vi "SetChainLength.vi"(8 "error in (no error)":errorcluster, 10 "Chain Length":u8, 11 "ControlState in":T1 {"ChainMask" format="0x%02x"}) -> (0 "error out":errorcluster, 3 "ControlState out":T1 {"ChainMask" format="0x%02x"})   [LabVIEW 2020, in "ArduinoSerialBling.lvlib"]
uses:
  ArduinoSerialBling.lvlib
  ControlState.ctl
  ChainState.ctl
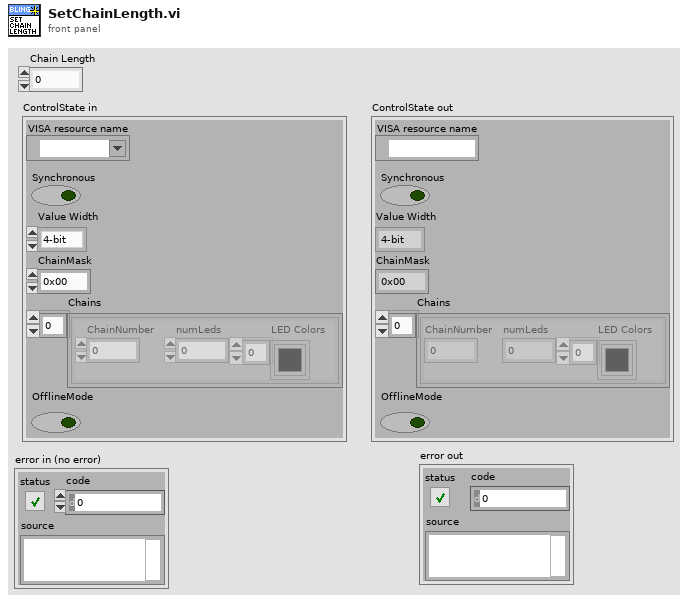
[diagram p1: front panel]
types:
  T1 = typedef "ArduinoSerialBling.lvlib/ControlState.ctl" = cluster{"VISA resource name":refnum<visa-resource-name>, "Synchronous":bool, "Value Width":enum16{"4-bit", "8-bit"}, "ChainMask":u8, "Chains":T2[], "OfflineMode":bool}
  T2 = typedef "ArduinoSerialBling.lvlib/ChainState.ctl" = cluster{"ChainNumber":u8, "numLeds":u8, "LED Colors":u32[]}
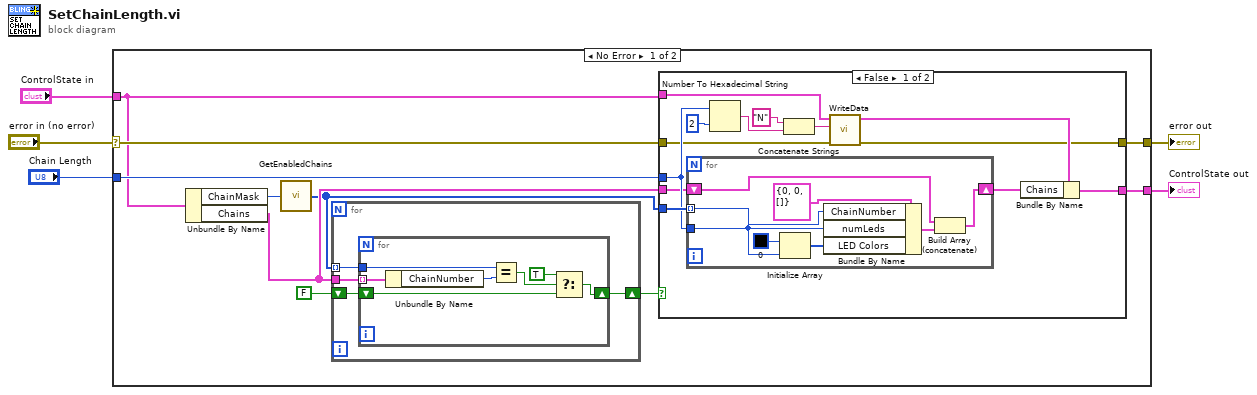
[diagram p0: block diagram]
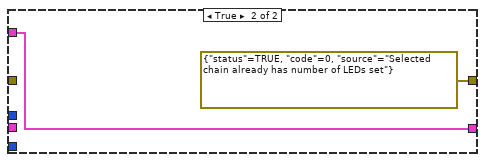
[diagram p2: hidden frame]
diagram:
  n1 = case shown="No Error" "error in (no error)" {
    selector: "error in (no error)" -> [w15 w50]
    tunnel: "ControlState in" -> [w11 w51]
    tunnel: [w10 w51] -> w5
    tunnel: [w14 w50] -> w2
    tunnel: "Chain Length" -> [w12 _]
    frame No Error {
      n2 = Unbundle By Name(w11) -> ("ChainMask"=w13:u8, "Chains"=w8:T2[])
      n3 = call "GetEnabledChains.vi"("ChainMask"=w13) -> ("Array"=w7:u8[])
      n4 = for {
        shift-right: [w16] -> w6
        shift-left: FALSE -> [w17]
        tunnel: w8 -> [w19]
        tunnel: w7 -> [w18] mode=indexing
        n5 = for {
          tunnel: w19 -> [w25] mode=indexing
          tunnel: w18 -> [w26]
          shift-right: [w20] -> w16
          shift-left: w17 -> [w22]
          n6 = Unbundle By Name(w25) -> ("ChainNumber"=w24:u8)
          n7 = Equal?(x=w26, y=w24) -> (x = y?=w23:bool)
          n8 = Select(t=TRUE, s=w23, f=w22) -> (s? t:f=w20:bool)
        }
      }
      n9 = case shown="False" w6 {
        tunnel: w15 -> [w28 _]
        tunnel: [w29 errorcluster {"status"=TRUE, "code"=0, "source"="Selected chain already has number of LEDs set"} ("error out")] -> w14
        tunnel: w7 -> [w36 _]
        tunnel: w12 -> [w35 _]
        tunnel: w8 -> [w34 _]
        tunnel: w11 -> [w31 w49]
        tunnel: [w32 w49] -> w10
        frame False {
          n10 = for {
            tunnel: w36 -> [w44] mode=indexing
            tunnel: w35 -> [w43]
            shift-right: [w40] -> w33
            shift-left: w34 -> [w42]
            n11 = Initialize Array(u32 0, w43) -> (w45:u32[])
            n12 = Bundle By Name(cluster=T2 {"ChainNumber"=0, "numLeds"=0, "LED Colors"=[]} ("ChainState"), "ChainNumber"=w44, "numLeds"=w43, "LED Colors"=w45) -> (w41:T2)
            n13 = Build Array (concatenate)(w42, w41) -> (w40:T2[])
          }
          n14 = Number To Hexadecimal String(1:i16 2 ("width (-)"), 2:w35) -> (0:w38:string)
          n15 = Concatenate Strings("N", w38) -> (w27:string)
          n16 = call "WriteData.vi"("error in (no error)"=w28, "Command"=w27, "ControlState in"=w31) -> ("error out"=w29:errorcluster, "ControlState out"=w30:T1)  [unwired: 5 in, 2 out]
          n17 = Bundle By Name(cluster=w30, "Chains"=w33) -> (w32:T1)
        }
        frame True {
        }
      }
    }
    frame Error {
    }
  }
  "ControlState out" <- w5
  "error out" <- w2
